vi "Zstack code with curved sawtooth.vi"() -> ()   [LabVIEW 2020]
uses:
  <vilib>/Analysis/1siggen.llb/Ramp Pattern by Samples.vi
  <vilib>/DAQmx/write.llb/DAQmx Write (Analog 1D Wfm NChan NSamp).vi
  <vilib>/DAQmx/create/channels.llb/DAQmx Create Channel (AO-Voltage-Basic).vi
  <vilib>/DAQmx/configure/timing.llb/DAQmx Timing (Use Waveform).vi
  <vilib>/DAQmx/miscellaneous.llb/DAQmx Fill In Error Info.vi
  <vilib>/measure/NI_MABase.lvlib
  <vilib>/Analysis/NI_AALBase.lvlib
panel:
  in  "Camera trigger delay (degrees)":dbl=5.0 format="%.2p"
  in  "Sawtooth Amplitude":dbl=-0.23
  in  "Sawtooth Offset":dbl=-0.004 format="%.2p"
  out "Waveform Graph 3":waveform(dbl)[](graph)=[{"t0"=timestamp(0 s since 1904-01-01), "dt"=0.001, "Y"=array[1000 elements]}, {"t0"=timestamp(0 s since 1904-01-01), "dt"=0.001, "Y"=array[1000 elements]}]
  out "# Samples written per channel":u32=1000
  in  "Stop Analog Signal":bool
  out "Error out":errorcluster
  in  "Disable Axis":bool
  in  "Exposure time (ms)":dbl=1000.0
  in  "Z step size (um)":dbl=0.2
  out "Number of Slices":dbl=100.0
  in  "Input will be multiplied by 5":dbl=20.0
  in  "Acquire Z Stack?":bool=TRUE
  out "GetFirmwareVersion 2":string="3.03\r"
  out "Connected":bool=TRUE
  in  "SPIIPLUSCOM660Lib.IAsyncChannel":refnum<k7>
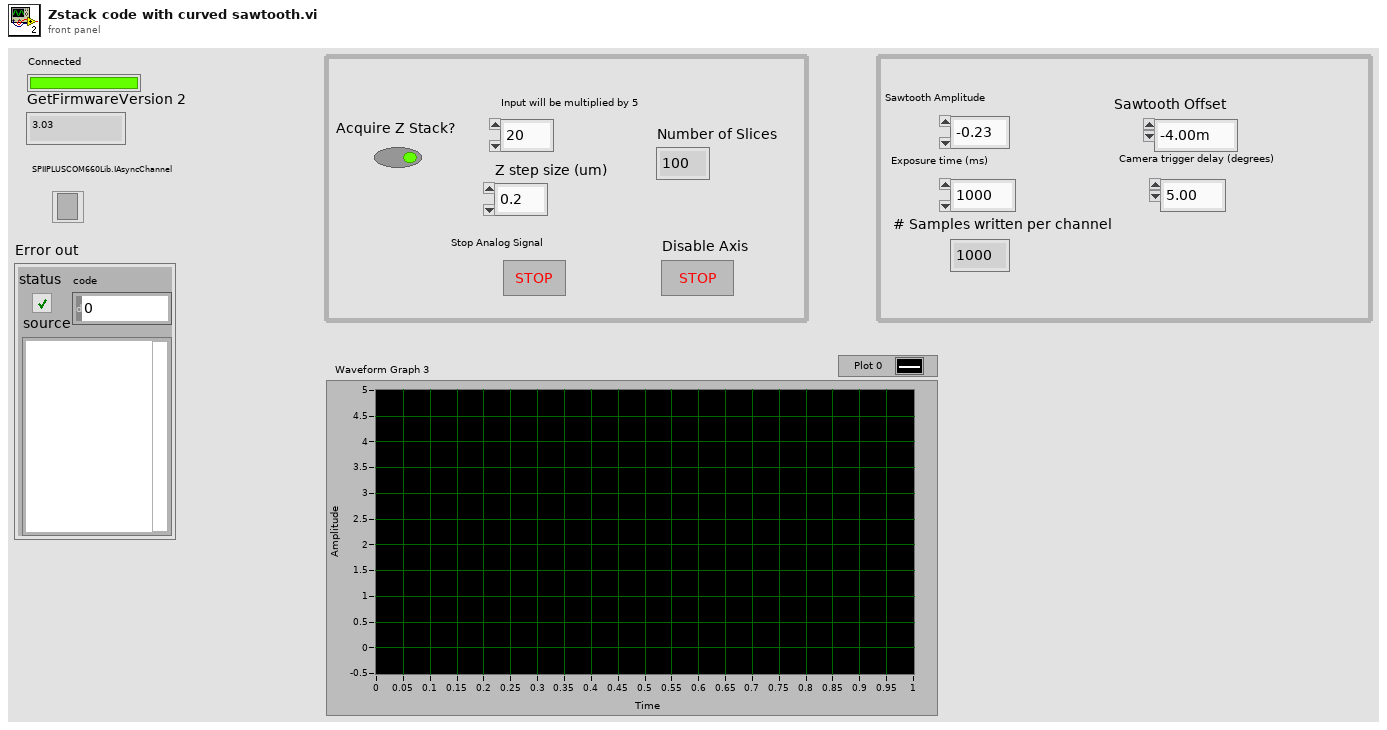
[diagram p1: front panel]
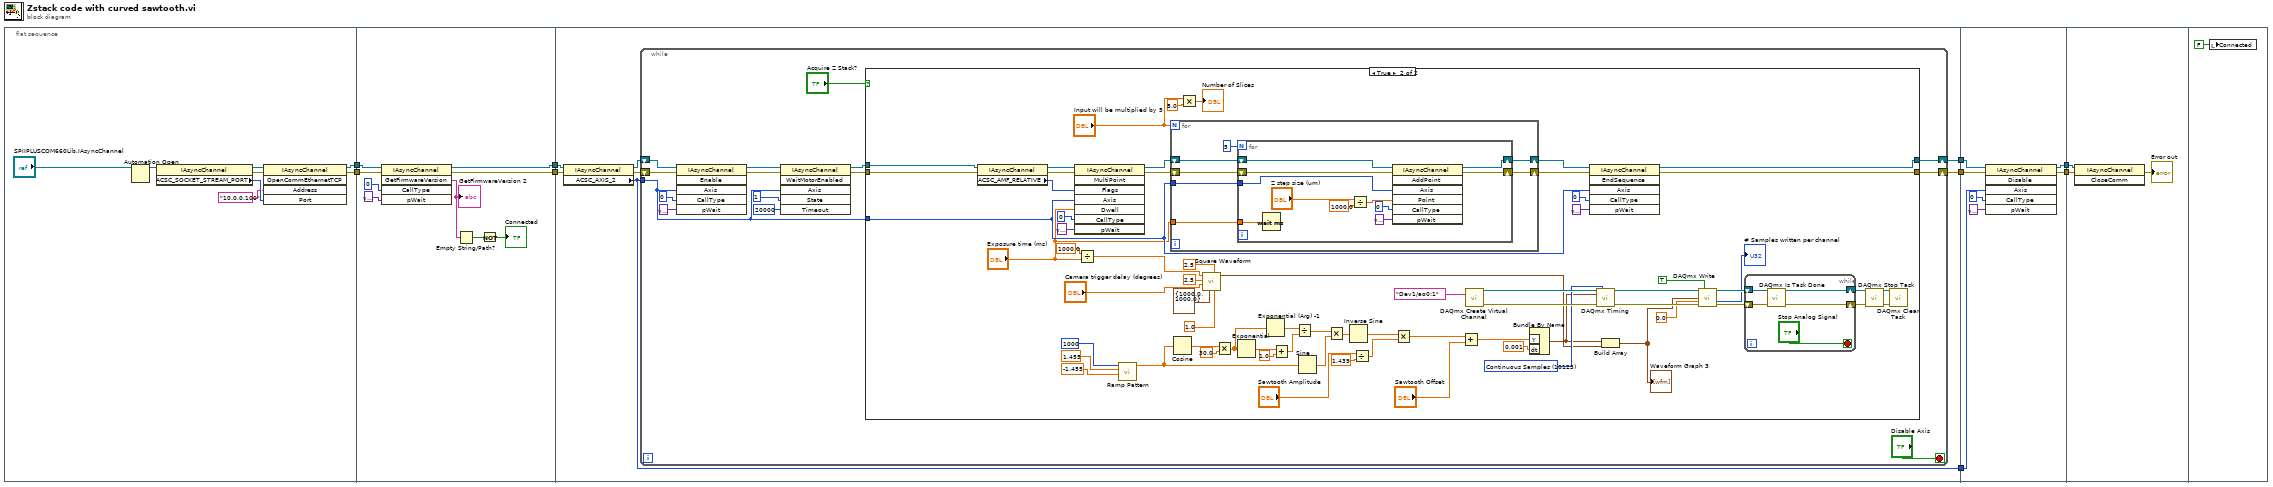
[diagram p0: block diagram]
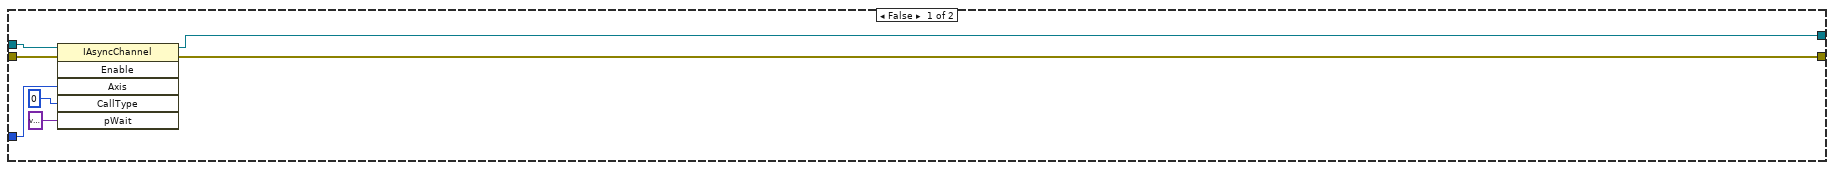
[diagram p2: hidden frame]
diagram:
  n1 = flat-sequence {
    tunnel: [w12] -> w9
    tunnel: [w11] -> w8
    tunnel: w9 -> [w22]
    tunnel: w8 -> [w21]
    tunnel: [w19] -> w7
    tunnel: [w18] -> w6
    tunnel: w7 -> [w31]
    tunnel: w6 -> [w30]
    tunnel: [w33] -> w5
    tunnel: [w32] -> w4
    tunnel: [w29] -> w3
    tunnel: w5 -> [w152]
    tunnel: w4 -> [w151]
    tunnel: [w150] -> w2
    tunnel: [w149] -> w1
    tunnel: w3 -> [w148]
    tunnel: w2 -> [w154]
    tunnel: w1 -> [w153]
    frame #0 {
      n2 = Automation Open(Automation Refnum="SPIIPLUSCOM660Lib.IAsyncChannel") -> (Automation Refnum=w17:refnum<k7>)  [unwired: 3 in, 1 out]
      n3 = property class="IAsyncChannel"(reference=w17) -> (reference out=w16:refnum<k7>, error out=w10:errorcluster, "ACSC_SOCKET_STREAM_PORT"=w14:i32)  [unwired: 1 in]
      n4 = invoke class="IAsyncChannel" method="OpenCommEthernetTCP"(reference=w16, error in=w10, "Address"="10.0.0.100", "Port"=w14) -> (reference out=w12:refnum<k7>, error out=w11:errorcluster)  [unwired: 1 in, 3 out]
    }
    frame #1 {
      n5 = invoke class="IAsyncChannel" method="GetFirmwareVersion"(reference=w22, error in=w21, "CallType"=u64 0, "pWait"=variant) -> (reference out=w19:refnum<k7>, error out=w18:errorcluster, "GetFirmwareVersion"=w24:string)  [unwired: 1 in, 2 out]
      "GetFirmwareVersion 2" <- w24
      n6 = Empty String/Path?(string/path=w24) -> (empty?=w23:bool)
      n7 = Not(x=w23) -> (.not. x?=→"Connected":bool)
    }
    frame #2 {
      n8 = property class="IAsyncChannel"(reference=w31, error in=w30) -> (reference out=w28:refnum<k7>, error out=w27:errorcluster, "ACSC_AXIS_2"=w29:i32)
      n9 = while {
        shift-right: [w48] -> w33
        shift-left: w28 -> [w40]
        shift-right: [w47] -> w32
        shift-left: w27 -> [w39]
        tunnel: w29 -> [w36]
        stop <- "Disable Axis" stop-if-true
        n10 = invoke class="IAsyncChannel" method="Enable"(reference=w40, error in=w39, "Axis"=w36, "CallType"=u64 0, "pWait"=variant) -> (reference out=w44:refnum<k7>, error out=w43:errorcluster)  [unwired: 1 in, 4 out]
        n11 = invoke class="IAsyncChannel" method="WaitMotorEnabled"(reference=w44, error in=w43, "Axis"=w36, "State"=1, "Timeout"=20000) -> (reference out=w35:refnum<k7>, error out=w34:errorcluster)  [unwired: 1 in, 4 out]
        n12 = case shown="True" "Acquire Z Stack?" {
          tunnel: w35 -> [w55 w110]
          tunnel: w34 -> [w54 w111]
          tunnel: [w53 w108] -> w48
          tunnel: [w52 w109] -> w47
          tunnel: w36 -> [w51 w107]
          frame False {
            n13 = invoke class="IAsyncChannel" method="Enable"(reference=w55, error in=w54, "Axis"=w51, "CallType"=u64 0, "pWait"=variant) -> (reference out=w53:refnum<k7>, error out=w52:errorcluster)  [unwired: 1 in, 4 out]
          }
          frame True {
            w98 = 10123 items=["Finite Samples"=10178, "Continuous Samples"=10123, "Hardware Timed Single Point"=12522] ("sample mode")
            n14 = property class="IAsyncChannel"(reference=w110, error in=w111) -> (reference out=w120:refnum<k7>, error out=w119:errorcluster, "ACSC_AMF_RELATIVE"=w116:i32)
            n15 = invoke class="IAsyncChannel" method="MultiPoint"(reference=w120, error in=w119, "Flags"=w116, "Axis"=w107, "Dwell"="Exposure time (ms)", "CallType"=u64 0, "pWait"=variant) -> (reference out=w115:refnum<k7>, error out=w114:errorcluster)  [unwired: 1 in, 6 out]
            n16 = Divide(x=1000.0, y="Exposure time (ms)") -> (x/y=w81:dbl)
            n17 = call-poly <vilib>:"Ramp Pattern.vi"("start"=-1.455, "end"=1.455, "samples"=1000) -> ("Ramp Pattern"=w63:dbl[])  [unwired: 7 in, 1 out]
            n18 = for {
              N: "Input will be multiplied by 5" -> [_]
              tunnel: w107 -> [w130]
              tunnel: "Exposure time (ms)" -> [w129]
              shift-right: [w132] -> w113
              shift-left: w115 -> [w134]
              shift-right: [w131] -> w112
              shift-left: w114 -> [w133]
              n19 = for {
                N: 5 -> [_]
                tunnel: w130 -> [w145]
                shift-right: [w140] -> w132
                shift-left: w134 -> [w144]
                shift-right: [w139] -> w131
                shift-left: w133 -> [w143]
                tunnel: w129 -> [w135]
                n20 = Wait (ms)(milliseconds to wait=w135) -> ()  [unwired: 1 out]
                n21 = Divide(x="Z step size (um)", y=1000.0) -> (x/y=w136:dbl)
                n22 = invoke class="IAsyncChannel" method="AddPoint"(reference=w144, error in=w143, "Axis"=w145, "Point"=w136, "CallType"=u64 0, "pWait"=variant) -> (reference out=w140:refnum<k7>, error out=w139:errorcluster)  [unwired: 1 in, 5 out]
              }
            }
            n23 = Cosine(x=w63) -> (cos(x)=w76:dbl[])
            n24 = Multiply(x="Input will be multiplied by 5", y=5.0) -> (x*y=→"Number of Slices":dbl)
            n25 = call <vilib>:"Square Waveform.vi"("duty cycle (%)"=1.0, "offset"=2.5, "sampling info"=cluster{"Fs":dbl, "#s":dbl} {"Fs"=1000.0, "#s"=1000.0}, "phase"="Camera trigger delay (degrees)", "amplitude"=2.5, "frequency"=w81) -> ("signal out"=w84:waveform(dbl))  [unwired: 4 in, 1 out]
            n26 = Multiply(x=w76, y=30.0) -> (x*y=w68:dbl[])
            n27 = Exponential(1:w68) -> (0:w71:dbl[])
            n28 = Exponential (Arg) -1(1:w68) -> (0:w75:dbl[])
            n29 = Add(x=w71, y=1.0) -> (x+y=w69:dbl[])
            n30 = Divide(x=w75, y=w69) -> (x/y=w74:dbl[])
            n31 = Sine(x=w63) -> (sin(x)=w73:dbl[])
            n32 = Multiply(x=w74, y=w73) -> (x*y=w72:dbl[])
            n33 = Inverse Sine(1:w72) -> (0:w65:dbl[])
            n34 = Divide(x="Sawtooth Amplitude", y=1.439) -> (x/y=w66:dbl)
            n35 = Multiply(x=w65, y=w66) -> (x*y=w62:dbl[])
            n36 = Add(x=w62, y="Sawtooth Offset") -> (x+y=w61:dbl[])
            n37 = call-poly <vilib>:"DAQmx Create Virtual Channel.vi"("physical channels"=tag "Dev1/ao0:1") -> ("task out"=w100:refnum<k21>, "error out"=w99:errorcluster)  [unwired: 13 in]
            n38 = Bundle By Name("Y"=w61, "dt"=0.001) -> (w60:waveform(dbl))  [unwired: 1 in]
            n39 = invoke class="IAsyncChannel" method="EndSequence"(reference=w113, error in=w112, "Axis"=w107, "CallType"=u64 0, "pWait"=variant) -> (reference out=w108:refnum<k7>, error out=w109:errorcluster)  [unwired: 1 in, 4 out]
            n40 = call-poly <vilib>:"DAQmx Timing.vi"("task/channels in"=w100, "sample mode"=w98, "waveform"=w60, "error in"=w99) -> ("task out"=w95:refnum<k21>, "error out"=w94:errorcluster)  [unwired: 10 in]
            n41 = Build Array(w60, w84) -> (w82:waveform(dbl)[])
            "Waveform Graph 3" <- w82
            n42 = call-poly <vilib>:"DAQmx Write.vi"("task/channels in"=w95, "auto start"=TRUE, "data"=w82, "timeout"=0.0, "error in"=w94) -> ("task out"=w96:refnum<k21>, "number of samples written per channel"=→"# Samples written per channel":u32, "error out"=w97:errorcluster)  [unwired: 8 in]
            n43 = while {
              shift-right: [w124] -> w92
              shift-left: w96 -> [w127]
              shift-right: [w125] -> w93
              shift-left: w97 -> [w126]
              stop <- "Stop Analog Signal" stop-if-true
              n44 = call <vilib>:"DAQmx Is Task Done.vi"("task/channels in"=w127, "error in"=w126) -> ("task out"=w124:refnum<k21>, "error out"=w125:errorcluster)  [unwired: 11 in, 1 out]
            }
            n45 = call <vilib>:"DAQmx Stop Task.vi"("task/channels in"=w92, "error in"=w93) -> ("task out"=w101:refnum<k21>, "error out"=w102:errorcluster)  [unwired: 12 in]
            n46 = call <vilib>:"DAQmx Clear Task.vi"("task in"=w101, "error in"=w102) -> ()  [unwired: 13 in, 1 out]
          }
        }
      }
    }
    frame #3 {
      n47 = invoke class="IAsyncChannel" method="Disable"(reference=w152, error in=w151, "Axis"=w148, "CallType"=u64 0, "pWait"=variant) -> (reference out=w150:refnum<k7>, error out=w149:errorcluster)  [unwired: 1 in, 4 out]
    }
    frame #4 {
      n48 = invoke class="IAsyncChannel" method="CloseComm"(reference=w154, error in=w153) -> (error out=→"Error out":errorcluster)  [unwired: 1 in, 2 out]
    }
    frame #5 {
      n49 = local write "Connected"(FALSE ("Connected")) -> ()
    }
  }
